vi "Get Min-Max Ranges.vi"(8 "error in (no error)":errorcluster, 11 "VISA resource name":refnum<visa-resource-name>) -> (0 "error out":errorcluster, 1 "I Max":dbl format="%_3e", 2 "V Max":dbl format="%_3e", 3 "VISA resource name out":refnum<visa-resource-name>, 4 "I Min":dbl format="%_3e", 5 "V Min":dbl format="%_3e")   [LabVIEW 2020, in "Keithley 2450.lvlib"]
doc: "Query returns the min and max voltage and current ranges on 2450/2460 SMU."
uses:
  Keithley 2450.lvlib
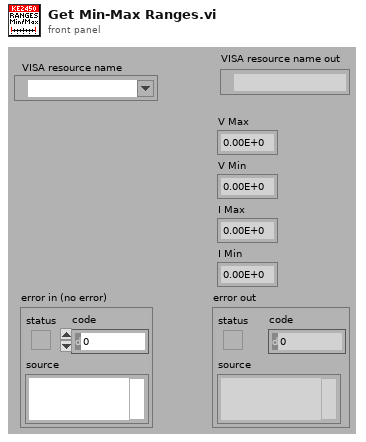
[diagram p1: front panel]
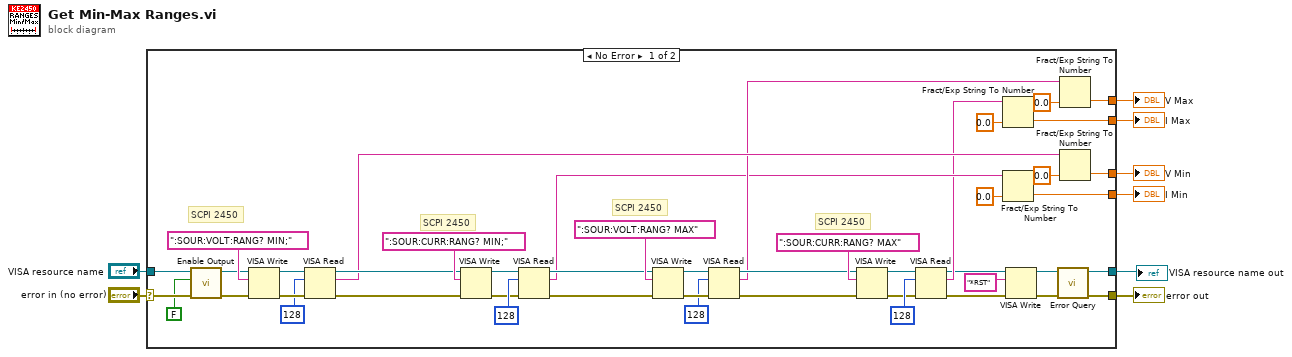
[diagram p0: block diagram]
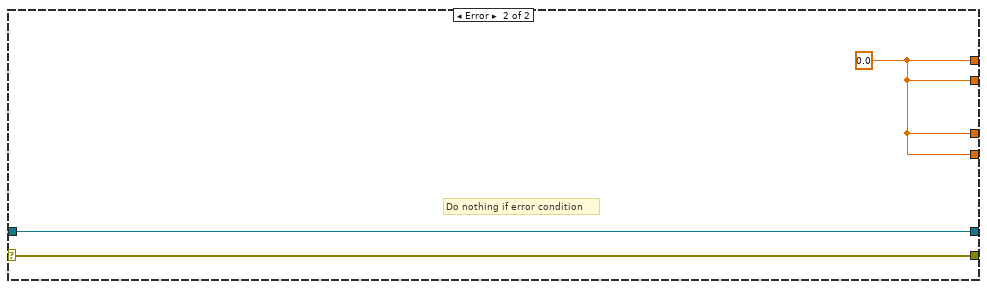
[diagram p2: hidden frame]
diagram:
  n1 = case shown="No Error" "error in (no error)" {
    selector: "error in (no error)" -> [w47 w57]
    tunnel: [w51 w57] -> w7
    tunnel: "VISA resource name" -> [w48 w56]
    tunnel: [w50 w56] -> w1
    tunnel: [w25 w55] -> w5
    tunnel: [w19 w55] -> w3
    tunnel: [w22 w55] -> w4
    tunnel: [w18 w55] -> w2
    frame No Error {
      # "SCPI 2450"
      # "SCPI 2450"
      # "SCPI 2450"
      # "SCPI 2450"
      n2 = call "Enable Output.vi"("error in (no error)"=w47, "Enable Output (T: Enable)"=FALSE, "VISA resource name"=w48) -> ("error out"=w45:errorcluster, "VISA resource name out"=w46:refnum<visa-resource-name>)  [unwired: 7 out]
      n3 = VISA Write(VISA resource name=w46, write buffer=":SOUR:VOLT:RANG? MIN;" ("format string"), error in (no error)=w45) -> (VISA resource name out=w53:refnum<visa-resource-name>, error out=w54:errorcluster)  [unwired: 1 out]
      n4 = VISA Read(VISA resource name=w53, byte count=u32 128, error in (no error)=w54) -> (VISA resource name out=w41:refnum<visa-resource-name>, read buffer=w17:string, error out=w40:errorcluster)  [unwired: 1 out]
      n5 = VISA Write(VISA resource name=w41, write buffer=":SOUR:CURR:RANG? MIN;", error in (no error)=w40) -> (VISA resource name out=w39:refnum<visa-resource-name>, error out=w38:errorcluster)  [unwired: 1 out]
      n6 = VISA Read(VISA resource name=w39, byte count=u32 128, error in (no error)=w38) -> (VISA resource name out=w26:refnum<visa-resource-name>, read buffer=w15:string, error out=w27:errorcluster)  [unwired: 1 out]
      n7 = VISA Write(VISA resource name=w26, write buffer=":SOUR:VOLT:RANG? MAX" ("format string"), error in (no error)=w27) -> (VISA resource name out=w36:refnum<visa-resource-name>, error out=w37:errorcluster)  [unwired: 1 out]
      n8 = VISA Read(VISA resource name=w36, byte count=u32 128, error in (no error)=w37) -> (VISA resource name out=w32:refnum<visa-resource-name>, read buffer=w16:string, error out=w31:errorcluster)  [unwired: 1 out]
      n9 = VISA Write(VISA resource name=w32, write buffer=":SOUR:CURR:RANG? MAX", error in (no error)=w31) -> (VISA resource name out=w30:refnum<visa-resource-name>, error out=w29:errorcluster)  [unwired: 1 out]
      n10 = VISA Read(VISA resource name=w30, byte count=u32 128, error in (no error)=w29) -> (VISA resource name out=w13:refnum<visa-resource-name>, read buffer=w14:string, error out=w11:errorcluster)  [unwired: 1 out]
      n11 = Fract/Exp String To Number(string=w14, default (0 dbl)=0.0 ("default (0 I32)")) -> (number=w22:dbl)  [unwired: 3 out]
      n12 = Fract/Exp String To Number(string=w15, default (0 dbl)=0.0 ("default (0 I32)")) -> (number=w18:dbl)  [unwired: 3 out]
      n13 = VISA Write(VISA resource name=w13, write buffer="*RST", error in (no error)=w11) -> (VISA resource name out=w12:refnum<visa-resource-name>, error out=w10:errorcluster)  [unwired: 1 out]
      n14 = call "Error Query.vi"("error in (no error)"=w10, "VISA resource name"=w12) -> ("error out"=w51:errorcluster, "VISA resource name out"=w50:refnum<visa-resource-name>)  [unwired: 8 out]
      n15 = Fract/Exp String To Number(string=w16, default (0 dbl)=0.0 ("default (0 I32)")) -> (number=w25:dbl)  [unwired: 3 out]
      n16 = Fract/Exp String To Number(string=w17, default (0 dbl)=0.0 ("default (0 I32)")) -> (number=w19:dbl)  [unwired: 3 out]
    }
    frame Error {
      w55 = 0.0
      # "Do nothing if error condition"
    }
  }
  "error out" <- w7
  "V Max" <- w5
  "I Max" <- w4
  "V Min" <- w3
  "I Min" <- w2
  "VISA resource name out" <- w1
